vi "ViresVTD.vi"(10 "Parameters":variant, 11 "Process":refnum<class "Process.lvclass">) -> ()   [LabVIEW 2023, in "Vires VTD Engine.lvlib"]
uses:
  Vires VTD Engine.lvlib
  <vilib>/NI/NIVS Inline Async API/_VS Inline Async API/Process/Process.lvclass
  Type/Status_Cluster.ctl
  Type/ConnectionStatus.ctl
  Type/CaseSelection.ctl
  Shared/Compiled.Settings.ctl
  System Explorer/RDB Data.ctl
  RDB/RDB Object.ctl
  RDB/RDB Player Object.ctl
  Shared/Network Settings.ctl
  Shared/Protocol.ctl
  Shared/SensorInfos.ctl
  Shared/SensorInfo.ctl
  Shared/Sensor Name.ctl
  MM/MM Data.ctl
  MM/MM Objects.ctl
  MM/MM Object.ctl
  Shared/Timedloop Settings.ctl
  <vilib>/NI/NIVS Inline Async API/_VS Inline Async API/Process/Process.lvclass/Process.ctl
  <vilib>/Platform/TimedLoop/XDataNode/timing_clust.ctl
  <vilib>/Platform/TimedLoop/XDataNode/nitl_modes.ctl
  <vilib>/Platform/TimedLoop/XDataNode/wakeup.ctl
  <vilib>/NI/NIVS Inline Async API/_Data Access Engine/Access Type Classes/Write/Write.lvclass/Write.ctl
  <vilib>/NI/NIVS Inline Async API/_Data Access Engine/Access Type Classes/Read/Read.lvclass/Read.ctl
  <vilib>/NI/NIVS Inline Async API/_Data Access Engine/Data Access Engine/Methods/Write.Data.vi
  <vilib>/NI/NIVS Inline Async API/_Data Access Engine/Data Access Engine/Methods/Read.Data.vi
  <vilib>/NI/NIVS Inline Async API/_VS Inline Async API/Process/Data Member Access/Read Data Access.vi
  <vilib>/NI/NIVS Inline Async API/_VS Inline Async API/Error Handling Process/SubVIs/Error.ConvertArray.vi
  <vilib>/NI/NIVS Inline Async API/_Data Access Engine/Access Type Classes/Write/Write.ProcessData.vi
  <vilib>/NI/NIVS Inline Async API/_Data Access Engine/Access Type Classes/Read/Read.ProcessData.vi
  <vilib>/NI/NIVS Inline Async API/_Data Access Engine/Access Type Classes/Write/Write.Buffer.vi
  <vilib>/NI/NIVS Inline Async API/_Data Access Engine/Access Type Classes/Write/Write.Commit.vi
  <vilib>/NI/NIVS Inline Async API/_Data Access Engine/Data Access Engine/Methods/ReadWrite.Lookup.vi
  <vilib>/NI/NIVS Inline Async API/_Data Access Engine/Data Access Engine/Methods/Write.Lookup.vi
  <vilib>/NI/NIVS Inline Async API/_Data Access Engine/Data Access Engine/Methods/Read.Lookup.vi
  <vilib>/NI/NIVS Inline Async API/_Data Access Engine/Data Access Engine/Data Access Engine.lvclass
  <vilib>/platform/TimedLoop/XDataNode/XDataNode.xnode
  RDB/RDB.lvlib
  Shared/Vires VTD Shared.lvlib
  MM/MM.lvlib
  SCP/SCP.lvlib
  <vilib>/Platform/TimedLoop/XDataNode/XDNodeRunTimeDep.lvlib
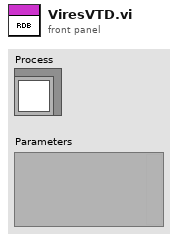
[diagram p1: front panel]
types:
  T1 = typedef "Vires VTD Engine.lvlib/Status_Cluster.ctl" = cluster{"simTime":dbl, "simFrame":dbl, "Connection Status":T2, "Connection Command":enum16{"Disconnect", "Connect"}, "Last Error":i32, "Case selection":T3}
  T2 = typedef "Vires VTD Engine.lvlib/ConnectionStatus.ctl" = enum16{"Disconnected", "Connected"}
  T3 = typedef "Vires VTD Engine.lvlib/CaseSelection.ctl" = enum32{"Idle", "Connecting", "Disconnecting", "Read/Write"}
  T4 = typedef "Vires VTD Shared.lvlib/Compiled.Settings.ctl" = cluster{"Name":string, "RDB Data Receive ":T5, "RDB Data Sent":T5, "vclient":path, "Network Settings":T8, "SensorInfos":T10, "mmanager":path, "Scenario Paths":string[], "Custom SCP Commands":string[], "Timed Loop Settings for TaskControl":T16, "Timed Loop Settings for ModuleManager":T16}
  T5 = typedef "Vires VTD Shared.lvlib/RDB Data.ctl" = T6[]
  T6 = typedef "RDB.lvlib/RDB Object.ctl" = cluster{"pkID":i32, "RDB Player Objects":T7[]}
  T7 = typedef "RDB.lvlib/RDB Player Object.ctl" = cluster{"PlayerID":i32, "Signals":string[], "adv para":i32}
  T8 = typedef "Vires VTD Shared.lvlib/Network Settings.ctl" = cluster{"IP adress":string, "RDB":cluster{"Protocol":T9, "Tx Port":u16, "Rx Port":u16, "Buffer Size":i32, "Timeout":u16}, "SCP":cluster{"Protocol":T9, "Tx Port":u16, "Rx Port":u16, "Buffer Size":i32, "Timeout":u16}}
  T9 = typedef "Vires VTD Shared.lvlib/Protocol.ctl" = enum16{"UDP", "TCP"}
  T10 = typedef "Vires VTD Shared.lvlib/SensorInfos.ctl" = T11[]
  T11 = typedef "Vires VTD Shared.lvlib/SensorInfo.ctl" = cluster{"Sensor Name":T12, "Protocol":T9, "Network port":i32, "# Culled Objects":i32, "PlayerID":u8, "MM Data":T13}
  T12 = typedef "Vires VTD Shared.lvlib/Sensor Name.ctl" = string
  T13 = typedef "Vires VTD Shared.lvlib/MM Data.ctl" = T14[]
  T14 = typedef "MM.lvlib/MM Objects.ctl" = cluster{"pkID":i32, "MM Objects":T15[]}
  T15 = typedef "MM.lvlib/MM Object.ctl" = cluster{"Object":i32, "Signals":string[]}
  T16 = typedef "Vires VTD Shared.lvlib/Timedloop Settings.ctl" = cluster{"Period(ms)":i64, "Priority":i32, "Processor":i32}
  T17 = typedef "Data Access Engine.lvlib/Data Access Engine.lvclass/ReadWrite.DVR.ctl" = refnum<data-value>
  T18 = typedef "Data Access Engine.lvlib/Data Access Engine.lvclass/Write.DVR.ctl" = refnum<data-value>
  T19 = typedef "Data Access Engine.lvlib/Data Access Engine.lvclass/Read.DVR.ctl" = refnum<data-value>
  T20 = typedef "RDB.lvlib/RDB References.ctl" = cluster{"RDB Receive Reference":T21, "RDB Send Reference":T21}
  T21 = typedef "RDB.lvlib/RDB Reference.ctl" = cluster{"Conversion References":refnum<k21>[], "RDB Data":T22[], "RDB Signals":dbl[], "noSignals":i32[]}
  T22 = typedef "XNET Frame FlexRay.ctl" = cluster{"timestamp":timestamp, "payload":u8[], "slot":u16, "type":T23, "cycle count":u8, "startup?":bool, "sync?":bool, "preamble?":bool, "ch A":bool, "ch B":bool, "echo?":bool}
  T23 = typedef "XNET Frame Type FlexRay.ctl" = u8
  T24 = typedef "Vires VTD Engine.lvlib/Settings.ctl" = cluster{"UDP Receiver":refnum<k16>, "UDP Sender":refnum<k16>, "Valid Packet":bool, "TCP":refnum<k5>, "Network Settings":T8, "vclient":path, "paeseHandle":u64, "builderHandle":u64}
  T25 = typedef "XDNodeRunTimeDep.lvlib/timing_clust.ctl" = cluster{"Expected End [f-1]":u64, "Actual End [f-1]":u64, "Finished Late? [f-1]":bool, "Expected End [i-1]":u64, "Actual End [i-1]":u64, "Finished Late? [i-1]":bool, "Expected Start [i]":u64, "Actual Start [i]":u64, "Expected Start [f]":u64, "Actual Start [f]":u64, "Source Name":string, "Structure Name":string, "Period":i64, "Deadline":i64, "Offset":i64, "Start":i64, "Priority":i32, "Timeout":i32, "Mode":T26, "Wakeup Reason":T27, "Error":errorcluster, "Source Type":string, "Secondary Source Type":string, "Global End Time":u64, "Global Start Time":u64, "Frame Duration":u64, "Iteration Duration":u64, "Assigned CPU":i32, "I/O Scan Engine Mode":u32}
  T26 = typedef "XDNodeRunTimeDep.lvlib/nitl_modes.ctl" = enum32{"No Change", "Process missed periods, maintain original phase", "Discard missed periods, maintain original phase", "Process missed periods, ignore original phase", "Discard missed periods, ignore original phase"}
  T27 = typedef "XDNodeRunTimeDep.lvlib/wakeup.ctl" = enum32{"Normal", "Aborted", "Asynchronous wakeup", "Timing source error", "Timed loop error", "Timeout"}
  T28 = typedef "SCP.lvlib/SCP_Cluster.ctl" = cluster{"SCP Command ":i32, "Custom SCP Command Index":i32, "Simulation Time":i32, "Step Size":i32, "Scenario Selection":i32, "Last SCP Error":i32, "Scenario Paths":string[], "Custom SCP Commands":string[]}
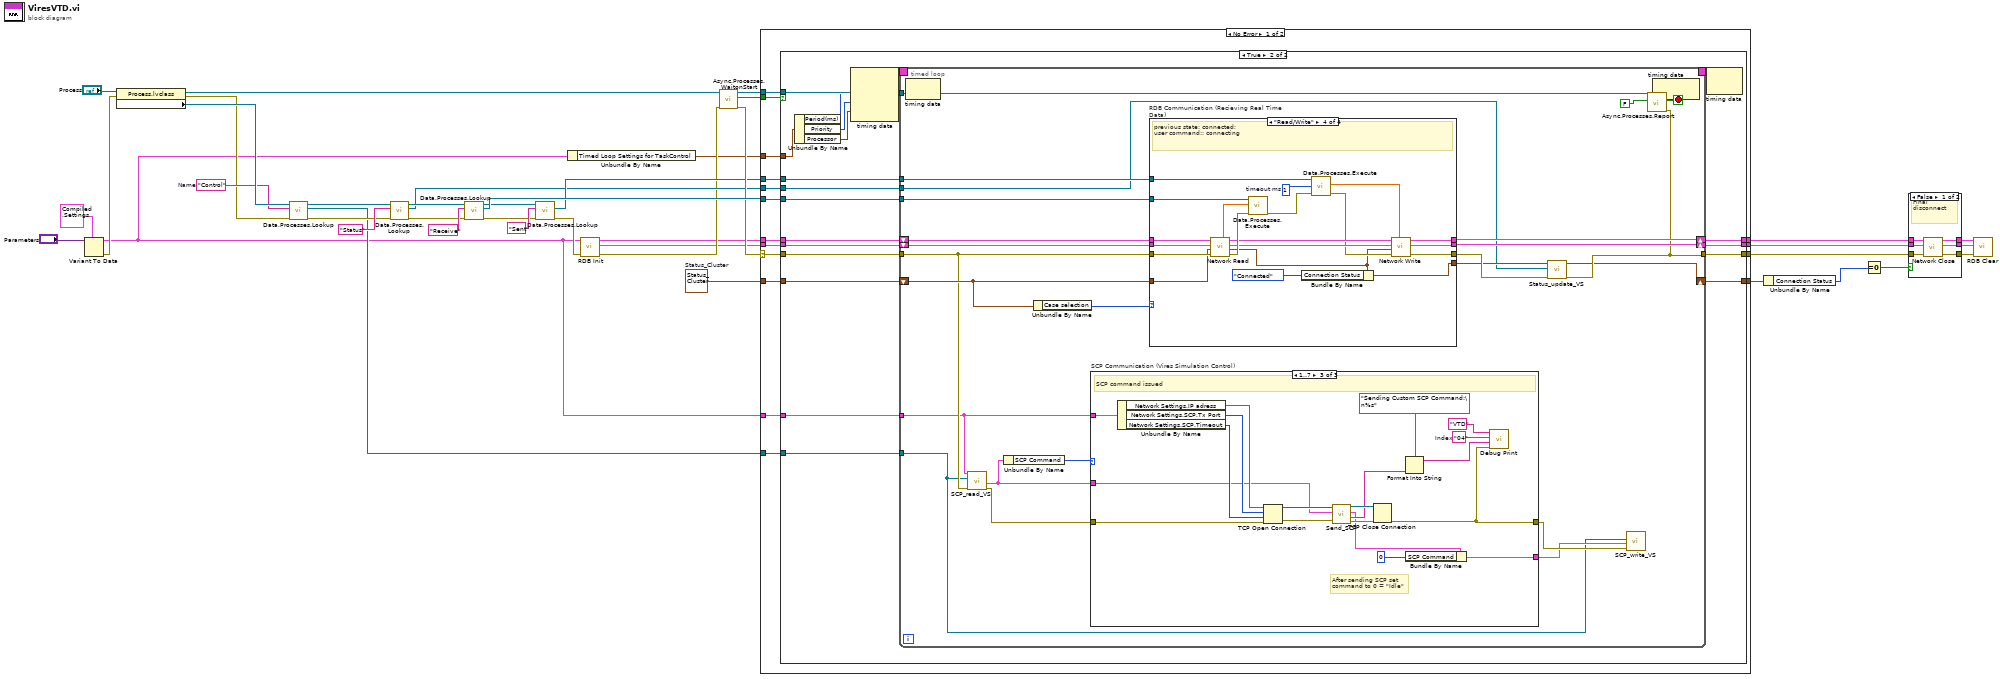
[diagram p0: block diagram]
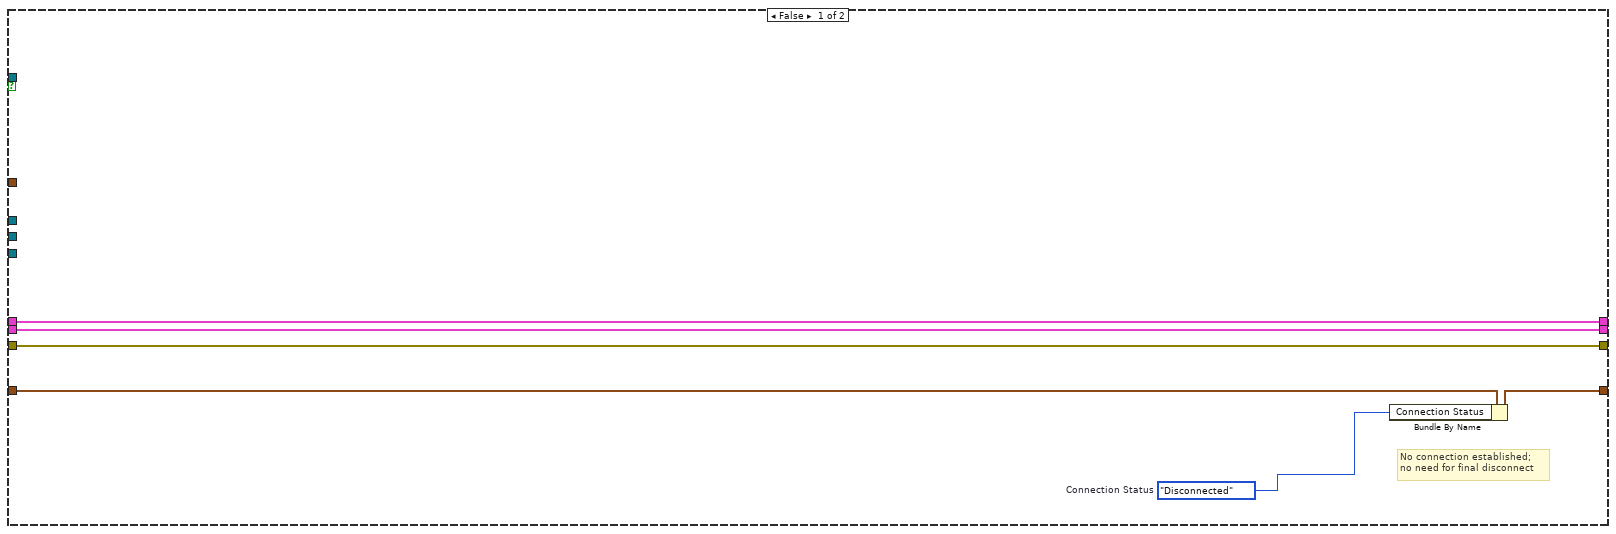
[diagram p2: hidden frame]
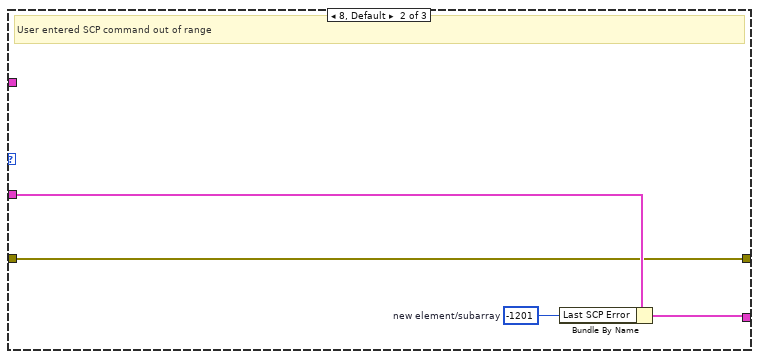
[diagram p4: hidden frame]
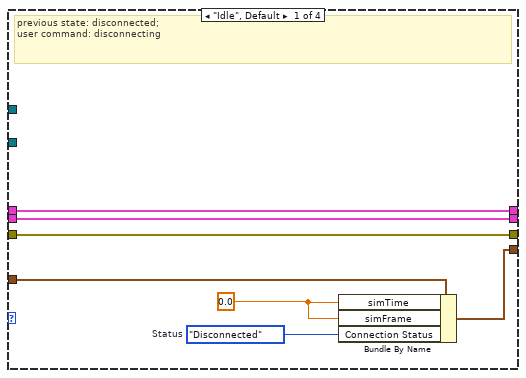
[diagram p5: hidden frame]
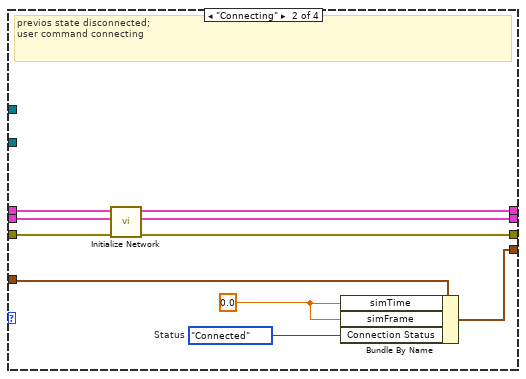
[diagram p6: hidden frame]
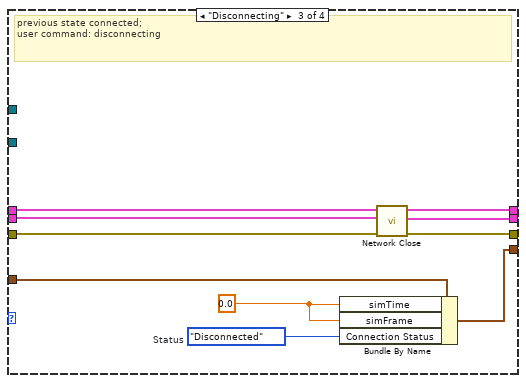
[diagram p7: hidden frame]
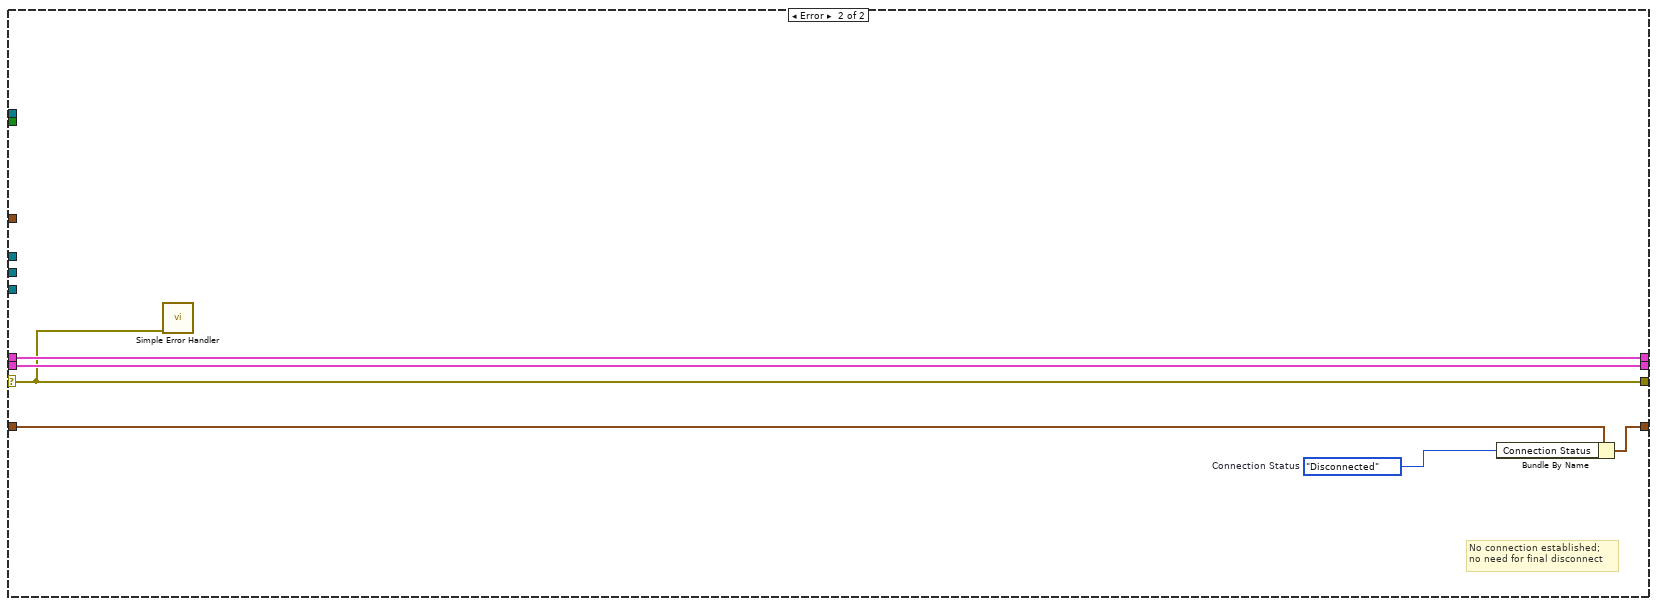
[diagram p8: hidden frame]
diagram:
  w4 = T1 {"simTime"=0.0, "simFrame"=0.0, "Connection Status"=enum."Disconnected", "Connection Command"=enum."Disconnect", "Last Error"=0, "Case selection"=enum."Connecting"}  # Status_Cluster
  w9 = "Control"  # Name
  n1 = Variant To Data(type=T4 {"Name"="", "RDB Data Receive "=[], "RDB Data Sent"=[], "vclient"=path "", "Network Settings"={"IP adress"="127.0.0.1", "RDB"={"Protocol"=enum."TCP", "Tx Port"=10, "Rx Port"=10, "Buffer Size"=204800, "Timeout"=10}, "SCP"={"Protocol"=enum."UDP", "Tx Port"=48190, "Rx Port"=48190, "Buffer Size"=204800, "Timeout"=10}}, "SensorInfos"=[], "mmanager"=path "", "Scenario Paths"=[], "Custom SCP Commands"=[], "Timed Loop Settings for TaskControl"={"Period(ms)"=2, "Priority"=100, "Processor"=-2}, "Timed Loop Settings for ModuleManager"={"Period(ms)"=2, "Priority"=100, "Processor"=-2}} ("Compiled.Settings"), Variant="Parameters") -> (data=w2:T4, error out=w23:errorcluster)  [unwired: 1 in]
  n2 = property class="Process.lvclass"(reference="Process", error in=w23) -> (reference out=w32:refnum<class "Process.lvclass">, error out=w7:errorcluster, "Data Member Access:Data Access"=w12:refnum<class "Data Access Engine.lvclass">)
  n3 = call-poly <vilib>:"Data.Processes.Lookup.vi"("error in (no error)"=w7, "Name"=w9, "Data Access API in"=w12) -> ("error out"=w10:errorcluster, "Ref"=w8:T17, "Data Access API out"=w11:refnum<class "Data Access Engine.lvclass">)  [unwired: 5 in, 1 out]
  n4 = call-poly <vilib>:"Data.Processes.Lookup.vi"("error in (no error)"=w10, "Name"="Status" ("Item Name"), "Data Access API in"=w11) -> ("error out"=w27:errorcluster, "Ref"=w24:T17, "Data Access API out"=w26:refnum<class "Data Access Engine.lvclass">)  [unwired: 5 in, 1 out]
  n5 = call-poly <vilib>:"Data.Processes.Lookup.vi"("error in (no error)"=w27, "Name"="Receive", "Data Access API in"=w26) -> ("error out"=w36:errorcluster, "Ref"=w35:T18, "Data Access API out"=w34:refnum<class "Data Access Engine.lvclass">)  [unwired: 5 in, 1 out]
  n6 = call-poly <vilib>:"Data.Processes.Lookup.vi"("error in (no error)"=w36, "Name"="Sent", "Data Access API in"=w34) -> ("error out"=w22:errorcluster, "Ref"=w28:T19)  [unwired: 5 in, 2 out]
  n7 = Unbundle By Name(w2) -> ("Timed Loop Settings for TaskControl"=w3:T16)
  n8 = call "RDB Init.vi"("error in"=w22, "Compiled.Settings"=w2) -> ("error out"=w21:errorcluster, "RDB References"=w20:T20, "Settings"=w1:T24)  [unwired: 7 in]
  n9 = call <vilib>:"Async.Processes.WaitonStart.vi"("error in (no error)"=w21, "Process"=w32) -> ("error out"=w30:errorcluster, "Execute"=w40:bool, "Process out"=w39:refnum<class "Process.lvclass">)  [unwired: 7 in]
  n10 = case shown="No Error" w30 {
    selector: w30 -> [w51 w190]
    tunnel: w40 -> [w56 _]
    tunnel: w39 -> [w55 _]
    tunnel: w35 -> [w54 _]
    tunnel: w1 -> [w53 w192]
    tunnel: w20 -> [w52 w191]
    tunnel: w28 -> [w50 _]
    tunnel: [w49 w192] -> w15
    tunnel: [w48 w191] -> w14
    tunnel: w24 -> [w47 _]
    tunnel: [w46 w190] -> w16
    tunnel: w8 -> [w45 _]
    tunnel: w2 -> [w44 _]
    tunnel: [w43 w189] -> w6
    tunnel: w4 -> [w42 w188]
    tunnel: w3 -> [w41 _]
    frame No Error {
      n11 = case shown="True" w56 {
        tunnel: w51 -> [w60 w73]
        tunnel: w55 -> [_ w75]
        tunnel: w54 -> [_ w82]
        tunnel: w53 -> [w62 w74]
        tunnel: w52 -> [w61 w81]
        tunnel: w50 -> [_ w80]
        tunnel: [w62 w79] -> w49
        tunnel: [w61 w78] -> w48
        tunnel: w47 -> [_ w77]
        tunnel: [w60 w76] -> w46
        tunnel: w45 -> [_ w72]
        tunnel: w44 -> [_ w71]
        tunnel: [w59 w70] -> w43
        tunnel: w42 -> [w58 w69]
        tunnel: w41 -> [_ w66]
        frame False {
          w57 = ConnectionStatus."Disconnected"  # Connection Status
          # "No connection established;\nno need for final disconnect"
          n12 = Bundle By Name(cluster=w58, "Connection Status"=w57) -> (w59:T1)
        }
        frame True {
          n13 = Unbundle By Name(w66) -> ("Period(ms)"=w65:i64, "Priority"=w64:i32, "Processor"=w63:i32)
          n14 = node-c288(w65, w64, w63) -> (w68:T25)  [unwired: 1 in]
          n15 = timed-loop {
            tunnel: w75 -> [w106]
            tunnel: w82 -> [w104]
            shift-right: [w100] -> w78
            shift-left: w81 -> [w103]
            tunnel: w80 -> [w101]
            shift-right: [w99] -> w79
            shift-left: w74 -> [w98]
            tunnel: w77 -> [w90]
            tunnel: w73 -> [w86]
            tunnel: [w93] -> w76
            tunnel: w72 -> [w84]
            tunnel: w71 -> [w83]
            shift-right: [w92] -> w70
            shift-left: w69 -> [w95]
            timing: w68 -> [_]
            timing-out: [_] -> w67
            stop <- w105 stop-if-true
            # "RDB Communication"
            n16 = node-c288() -> ()  [unwired: 1 in, 1 out]
            n17 = call "SCP_read_VS.vi"("error_in"=w86, "Ref"=w84, "Compiled.Settings"=w83) -> ("error_out"=w85:errorcluster, "SCP_Cluster_out"=w87:T28)  [unwired: 7 in]
            n18 = Unbundle By Name(w87) -> ("SCP Command"=w97:i32)
            n19 = Unbundle By Name(w95) -> ("Case selection"=w96:T3)
            n20 = case "SCP Communication (Vires Simulation Control)" shown="1..7" w97 {
              tunnel: [w109 w111 w121] -> w89
              tunnel: w85 -> [w109 w111 w120]
              tunnel: w83 -> [_ _ w119]
              tunnel: w87 -> [w110 w114 w118]
              tunnel: [w110 w112 w115] -> w88
              frame 0 {
                # "no SCP command issued;\nupdate VS UI"
              }
              frame 8, Default {
                w113 = -1201  # new element/subarray
                # "User entered SCP command out of range"
                n21 = Bundle By Name(cluster=w114, "Last SCP Error"=w113) -> (w112:T28)
              }
              frame 1..7 {
                w126 = "04"  # Index
                # "After sending SCP set\ncommand to 0 = \"Idle\""
                # "SCP command issued"
                n22 = Unbundle By Name(w119) -> ("Network Settings.IP adress"=w132:string, "Network Settings.SCP.Tx Port"=w131:u16, "Network Settings.SCP.Timeout"=w130:u16)
                n23 = TCP Open Connection(address=w132, remote port or service name=w131, timeout ms (60000)=w130, error in (no error)=w120) -> (connection ID=w129:refnum<k5>, error out=w133:errorcluster)  [unwired: 1 in]
                n24 = call "Send_SCP.vi"("error in (no error)"=w133, "SCP_Cluster_In"=w118, "TCP Network Connection in"=w129) -> ("error out"=w128:errorcluster, "CMD Msg"=w122:string, "SCP_Cluster_Out"=w117:T28, "TCP Network Connection out"=w127:refnum<k5>)  [unwired: 5 in]
                n25 = TCP Close Connection(connection ID=w127, error in (no error)=w128) -> (error out=w121:errorcluster)  [unwired: 1 in, 1 out]
                n26 = Format Into String(format string="Sending Custom SCP Command:\n%s", w122) -> (resulting string=w123:string)  [unwired: 2 in, 1 out]
                n27 = Bundle By Name(cluster=w117, "SCP Command"=0) -> (w115:T28)
                n28 = call "Debug Print.vi"("error out"=w121, "comment"=w123, "Index"=w126, "Module"="VTD") -> ()  [unwired: 8 in]
              }
            }
            n29 = case "RDB Communication (Recieving Real Time Data)" shown="\"Read/Write\"" w96 {
              tunnel: w104 -> [_ _ _ w180]
              tunnel: w98 -> [w140 w149 w157 w179]
              tunnel: w103 -> [w139 w148 w156 w178]
              tunnel: w86 -> [w138 w150 w155 w177]
              tunnel: w101 -> [_ _ _ w176]
              tunnel: [w139 w146 w159 w175] -> w100
              tunnel: [w140 w147 w160 w174] -> w99
              tunnel: [w138 w145 w158 w173] -> w94
              tunnel: w95 -> [w137 w142 w152 w164]
              tunnel: [w134 w141 w151 w162] -> w91
              frame "Idle", Default {
                w136 = 0.0
                w135 = ConnectionStatus."Disconnected"  # Status
                # "previous state: disconnected; \nuser command: disconnecting"
                n30 = Bundle By Name(cluster=w137, "simTime"=w136, "simFrame"=w136, "Connection Status"=w135) -> (w134:T1)
              }
              frame "Connecting" {
                w144 = 0.0
                w143 = ConnectionStatus."Connected"  # Status
                # "previos state disconnected; \nuser command connecting"
                n31 = call "Initialize Network.vi"("error in (no error)"=w150, "RDB References"=w148, "Settings"=w149) -> ("error out"=w145:errorcluster, "RDB References"=w146:T20, "Settings"=w147:T24)  [unwired: 6 in]
                n32 = Bundle By Name(cluster=w142, "simTime"=w144, "simFrame"=w144, "Connection Status"=w143) -> (w141:T1)
              }
              frame "Disconnecting" {
                w154 = 0.0
                w153 = ConnectionStatus."Disconnected"  # Status
                # "previous state connected; \nuser command: disconnecting"
                n33 = Bundle By Name(cluster=w152, "simTime"=w154, "simFrame"=w154, "Connection Status"=w153) -> (w151:T1)
                n34 = call "Network Close.vi"("error in (no error)"=w155, "RDB References"=w156, "Settings"=w157) -> ("error out"=w158:errorcluster, "RDB References"=w159:T20, "Settings"=w160:T24)  [unwired: 6 in]
              }
              frame "Read/Write" {
                w170 = 1  # timeout ms
                # "previous state: connected; \nuser command:: connecting"
                n35 = call "Network Read.vi"("error in (no error)"=w177, "Status_Cluster_in"=w164, "RDB References in"=w178, "Settings"=w179) -> ("error out"=w172:errorcluster, "Status_Cluster_out"=w161:T1, "RDB References out"=w167:T20, "Settings"=w169:T24, "RDB Receive Reference.RDB Signals"=w171:dbl[])  [unwired: 2 in, 1 out]
                n36 = call-poly <vilib>:"Data.Processes.Execute.vi"("error in (no error)"=w172, "Values"=w171, "Ref"=w180) -> ("error out"=w165:errorcluster)  [unwired: 8 in]
                n37 = Bundle By Name(cluster=w161, "Connection Status"=ConnectionStatus."Connected") -> (w162:T1)
                n38 = call-poly <vilib>:"Data.Processes.Execute.vi"("error in (no error)"=w165, "timeout ms"=w170, "Ref"=w176) -> ("error out"=w166:errorcluster, "Values"=w168:dbl[])  [unwired: 6 in, 1 out]
                n39 = call "Network Write.vi"("Values"=w168, "error in (no error)"=w166, "Status_Cluster"=w161, "RDB References in"=w167, "Settings"=w169) -> ("error out"=w173:errorcluster, "RDB Reference out"=w175:T20, "Settings"=w174:T24)  [unwired: 4 in]
              }
            }
            n40 = call "Status_update_VS.vi"("error in (no error)"=w94, "Data Value Reference in"=w90, "Status_Cluster_out in"=w91) -> ("error out"=w93:errorcluster, "Status_Cluster_out out"=w92:T1)  [unwired: 7 in]
            n41 = call "SCP_write_VS.vi"("error_in"=w89, "SCP_Cluster_in"=w88, "Ref"=w84) -> ()  [unwired: 7 in, 2 out]
            n42 = call <vilib>:"Async.Processes.Report.vi"("Error"=w93, "Stop Async on Error?"=FALSE, "Process in"=w106) -> ("Stop"=w105:bool)  [unwired: 7 in, 1 out]
            n43 = node-c288() -> ()  [unwired: 1 in, 1 out]
          }
          n44 = node-c288(w67) -> ()  [unwired: 1 out]
        }
      }
    }
    frame Error {
      w187 = ConnectionStatus."Disconnected"  # Connection Status
      # "No connection established;\nno need for final disconnect"
      n45 = call <vilib>:"Simple Error Handler.vi"("error in (no error)"=w190) -> ()  [unwired: 4 in, 5 out]
      n46 = Bundle By Name(cluster=w188, "Connection Status"=w187) -> (w189:T1)
    }
  }
  n47 = Unbundle By Name(w6) -> ("Connection Status"=w5:T2)
  n48 = Equal To 0?(x=w5) -> (x = 0?=w13:bool)
  n49 = case shown="False" w13 {
    tunnel: [w198 w201] -> w19
    tunnel: [w197 w200] -> w18
    tunnel: [w196 w199] -> w17
    tunnel: w16 -> [w195 w199]
    tunnel: w15 -> [w194 w201]
    tunnel: w14 -> [w193 w200]
    frame False {
      # "Final disconnect"
      n50 = call "Network Close.vi"("error in (no error)"=w195, "RDB References"=w193, "Settings"=w194) -> ("error out"=w196:errorcluster, "RDB References"=w197:T20, "Settings"=w198:T24)  [unwired: 6 in]
    }
    frame True {
      # "Already disconnected"
    }
  }
  n51 = call "RDB Clear.vi"("error in (no error)"=w17, "RDB References"=w18, "Settings"=w19) -> ()  [unwired: 8 in, 1 out]
